vi "Refresh DTCs Event.vi"(0 "connection info":T1, 1 "Addresses":refnum<vi>, 2 "DTCs":refnum<vi>, 5 "State Variables":T3, 7 "Address Lookup Table":variant, 9 "To Top (T)":bool=TRUE, 12 "Error Q":refnum<queue>, 13 "VI Ref":refnum<vi>) -> (4 "connection info":T1, 8 "Address Lookup Table Out":variant)   [LabVIEW 2019, in "J1939 Addon Shared.lvlib"]
uses:
  J1939 Addon Shared.lvlib
  Types/Error Cluster.ctl
  Types/Error Types.ctl
  Types/Private Data.ctl
  <vilib>/NI/STM/TCP/TCP Connection Info.ctl
  <vilib>/NI/STM/SubVIs/MetaDataElement.ctl
  <vilib>/NI/STM/NI STM.lvlib
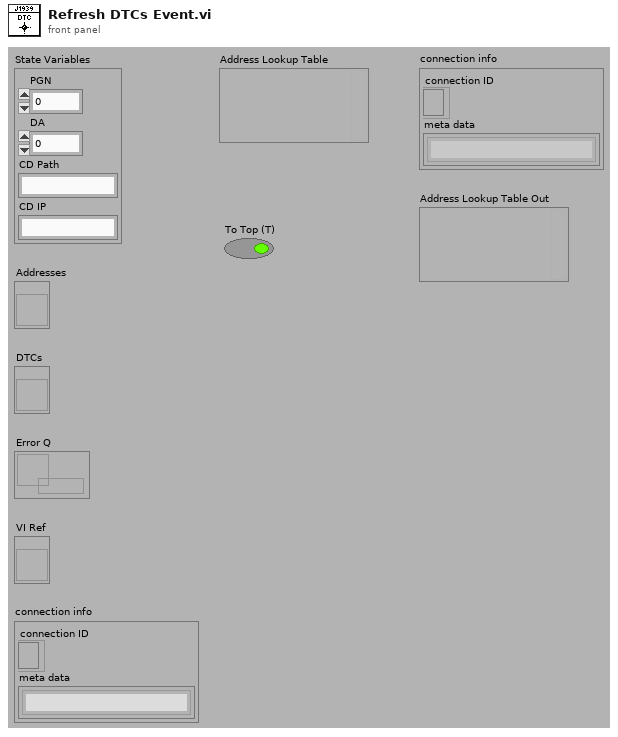
[diagram p1: front panel]
types:
  T1 = typedef "NI STM.lvlib/TCP Connection Info.ctl" = cluster{"connection ID":refnum<k5>, "meta data":T2[]}
  T2 = typedef "NI STM.lvlib/MetaDataElement.ctl" = string
  T3 = typedef "J1939 Addon Shared.lvlib/Private Data.ctl" = cluster{"PGN":u32, "DA":u8, "CD Path":string, "CD IP":string}
  T4 = typedef "J1939 Addon Shared.lvlib/Error Cluster.ctl" = cluster{"error out":errorcluster, "Enum":T5, "Address":u8, "Timestamp":timestamp}
  T5 = typedef "J1939 Addon Shared.lvlib/Error Types.ctl" = enum16{"Request", "RAW Generation", "Clear Active DTCs", "Clear Previous DTCs", "Addresses", "TLAs", "Get Active DTCs", "Get Previous DTCs", "TCP Connection"}
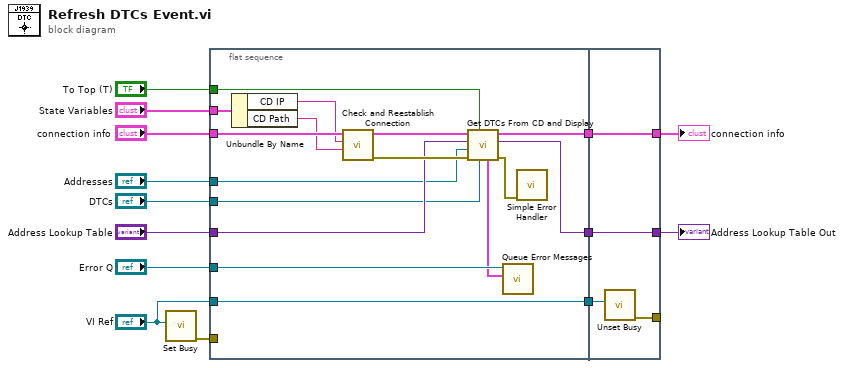
[diagram p0: block diagram]
diagram:
  n1 = call <vilib>:"Set Busy.vi"("VI reference (current VI)"="VI Ref") -> ("error out"=w7:errorcluster)  [unwired: 9 in, 1 out]
  n2 = flat-sequence {
    tunnel: [w26] -> w14
    tunnel: [w25] -> w13
    tunnel: "connection info" -> [w30]
    tunnel: "Address Lookup Table" -> [w27]
    tunnel: "State Variables" -> [w24]
    tunnel: w7 -> [_]
    tunnel: "Error Q" -> [w23]
    tunnel: "Addresses" -> [w18]
    tunnel: "DTCs" -> [w17]
    tunnel: [w16] -> w12
    tunnel: "VI Ref" -> [w16]
    tunnel: "To Top (T)" -> [w15]
    tunnel: [w33] -> w5
    tunnel: [w34] -> w4
    tunnel: w14 -> [w34]
    tunnel: w13 -> [w33]
    tunnel: [w32] -> _
    tunnel: w12 -> [w31]
    frame #0 {
      n3 = Unbundle By Name(w24) -> ("CD IP"=w19:string, "CD Path"=w20:string)
      n4 = call "Check and Reestablish Connection.vi"("CD Path"=w20, "IP Address"=w19, "connection info"=w30) -> ("error out"=w28:errorcluster, "connection info"=w29:T1)  [unwired: 7 in]
      n5 = call "Get DTCs From CD and Display.vi"("DTCs"=w17, "To Top (T)"=w15, "error in (no error)"=w28, "Addresses"=w18, "Lookup Table In"=w27, "connection info"=w29) -> ("error out"=w22:errorcluster, "Lookup Table Out"=w26:variant, "connection info"=w25:T1, "Error Array"=w21:T4[])  [unwired: 2 in]
      n6 = call "Queue Error Messages.vi"("Error Array"=w21, "queue out"=w23) -> ()  [unwired: 9 in, 1 out]
      n7 = call <vilib>:"Simple Error Handler.vi"("error in (no error)"=w22) -> ()  [unwired: 4 in, 5 out]
    }
    frame #1 {
      n8 = call <vilib>:"Unset Busy.vi"("VI reference (current VI)"=w31) -> ("error out"=w32:errorcluster)  [unwired: 10 in]
    }
  }
  "connection info" <- w5
  "Address Lookup Table Out" <- w4
